vi "Handle UNREGISTERED.vi"(8 "error in (no error)":errorcluster, 9 "WAMP Message":T16 {"Message Codes" items=["HELLO"=1, "WELCOME"=2, "ABORT"=3, "GOODBYE"=6, "ERROR"=8, "PUBLISH"=16, "PUBLISHED"=17, "SUBSCRIBE"=32, "SUBSCRIBED"=33, "UNSUBSCRIBE"=34, "UNSUBSCRIBED"=35, "EVENT"=36, "CALL"=48, "RESULT"=59, "REGISTER"=64, "REGISTERED"=65, "UNREGISTER"=66, "UNREGISTERED"=67, "INVOCATION"=68, "YIELD"=70]}, 10 "Message loop data (in)":T1, 11 "reference":refnum<class "WAMP Client.lvclass">) -> (0 "error out":errorcluster, 2 "Message Loop Data (Out)":T1, 3 "reference out":refnum<class "WAMP Client.lvclass">)   [LabVIEW 2020, in "wamplv.lvlib" / "WAMP Client.lvclass"]
uses:
  <vilib>/samangh/wamplv/WAMP Client/WAMP Client.lvclass
  <vilib>/samangh/wamplv/WAMP Client/TypeDef/WAMP Received Message.ctl
  <vilib>/samangh/wamplv/WAMP Message Codes.ctl
  <vilib>/samangh/wamplv/WAMP Client/TypeDef/Message Loop Shift Reg Data.ctl
  <vilib>/samangh/wamplv/WAMP Client/TypeDef/REGISTER Request Data.ctl
  <vilib>/samangh/wamplv/WAMP Client/TypeDef/Success or error.ctl
  <vilib>/samangh/wamplv/WAMP Client/TypeDef/Combined error.ctl
  <vilib>/samangh/wamplv/WAMP Client/TypeDef/WAMP Error Payload.ctl
  <vilib>/samangh/wamplv/WAMP Client/TypeDef/INVOCATION payload.ctl
  <vilib>/samangh/wamplv/WAMP Client/TypeDef/Publish Requests Map.ctl
  <vilib>/samangh/wamplv/WAMP Client/TypeDef/PUBLISH Request Data.ctl
  <vilib>/samangh/wamplv/WAMP Client/TypeDef/PUBLISH Result.ctl
  <vilib>/samangh/wamplv/WAMP Client/TypeDef/Endpoint Data.ctl
  <vilib>/samangh/wamplv/WAMP Client/TypeDef/CALL Request Map.ctl
  <vilib>/samangh/wamplv/WAMP Client/TypeDef/CALL Request Data.ctl
  <vilib>/samangh/wamplv/WAMP Client/TypeDef/RESULT Payload.ctl
  <vilib>/samangh/wamplv/WAMP Client/TypeDef/SUBSCRIBE Requests Map.ctl
  <vilib>/samangh/wamplv/WAMP Client/TypeDef/SUBSCRIBE Request Data.ctl
  <vilib>/samangh/wamplv/WAMP Client/TypeDef/Subscribe Result.ctl
  <vilib>/samangh/wamplv/WAMP Client/TypeDef/Event Payload.ctl
  <vilib>/samangh/wamplv/WAMP Client/TypeDef/Subscriptions Map.ctl
  <vilib>/samangh/wamplv/WAMP Client/TypeDef/Subscription Details.ctl
  <vilib>/samangh/wamplv/WAMP Client/TypeDef/Unsubscribe Requests Map.ctl
  <vilib>/samangh/wamplv/WAMP Client/TypeDef/UNSUBSCRIBE Request Data.ctl
  <vilib>/samangh/wamplv/WAMP Client/TypeDef/UNSUBSCRIBE Result.ctl
  <vilib>/samangh/wamplv/WAMP Client/TypeDef/Unregister requests map.ctl
  <vilib>/samangh/wamplv/WAMP Client/TypeDef/Unregister request.ctl
  <vilib>/samangh/wamplv/WAMP Client/WAMP Client.lvclass/WAMP Client.ctl
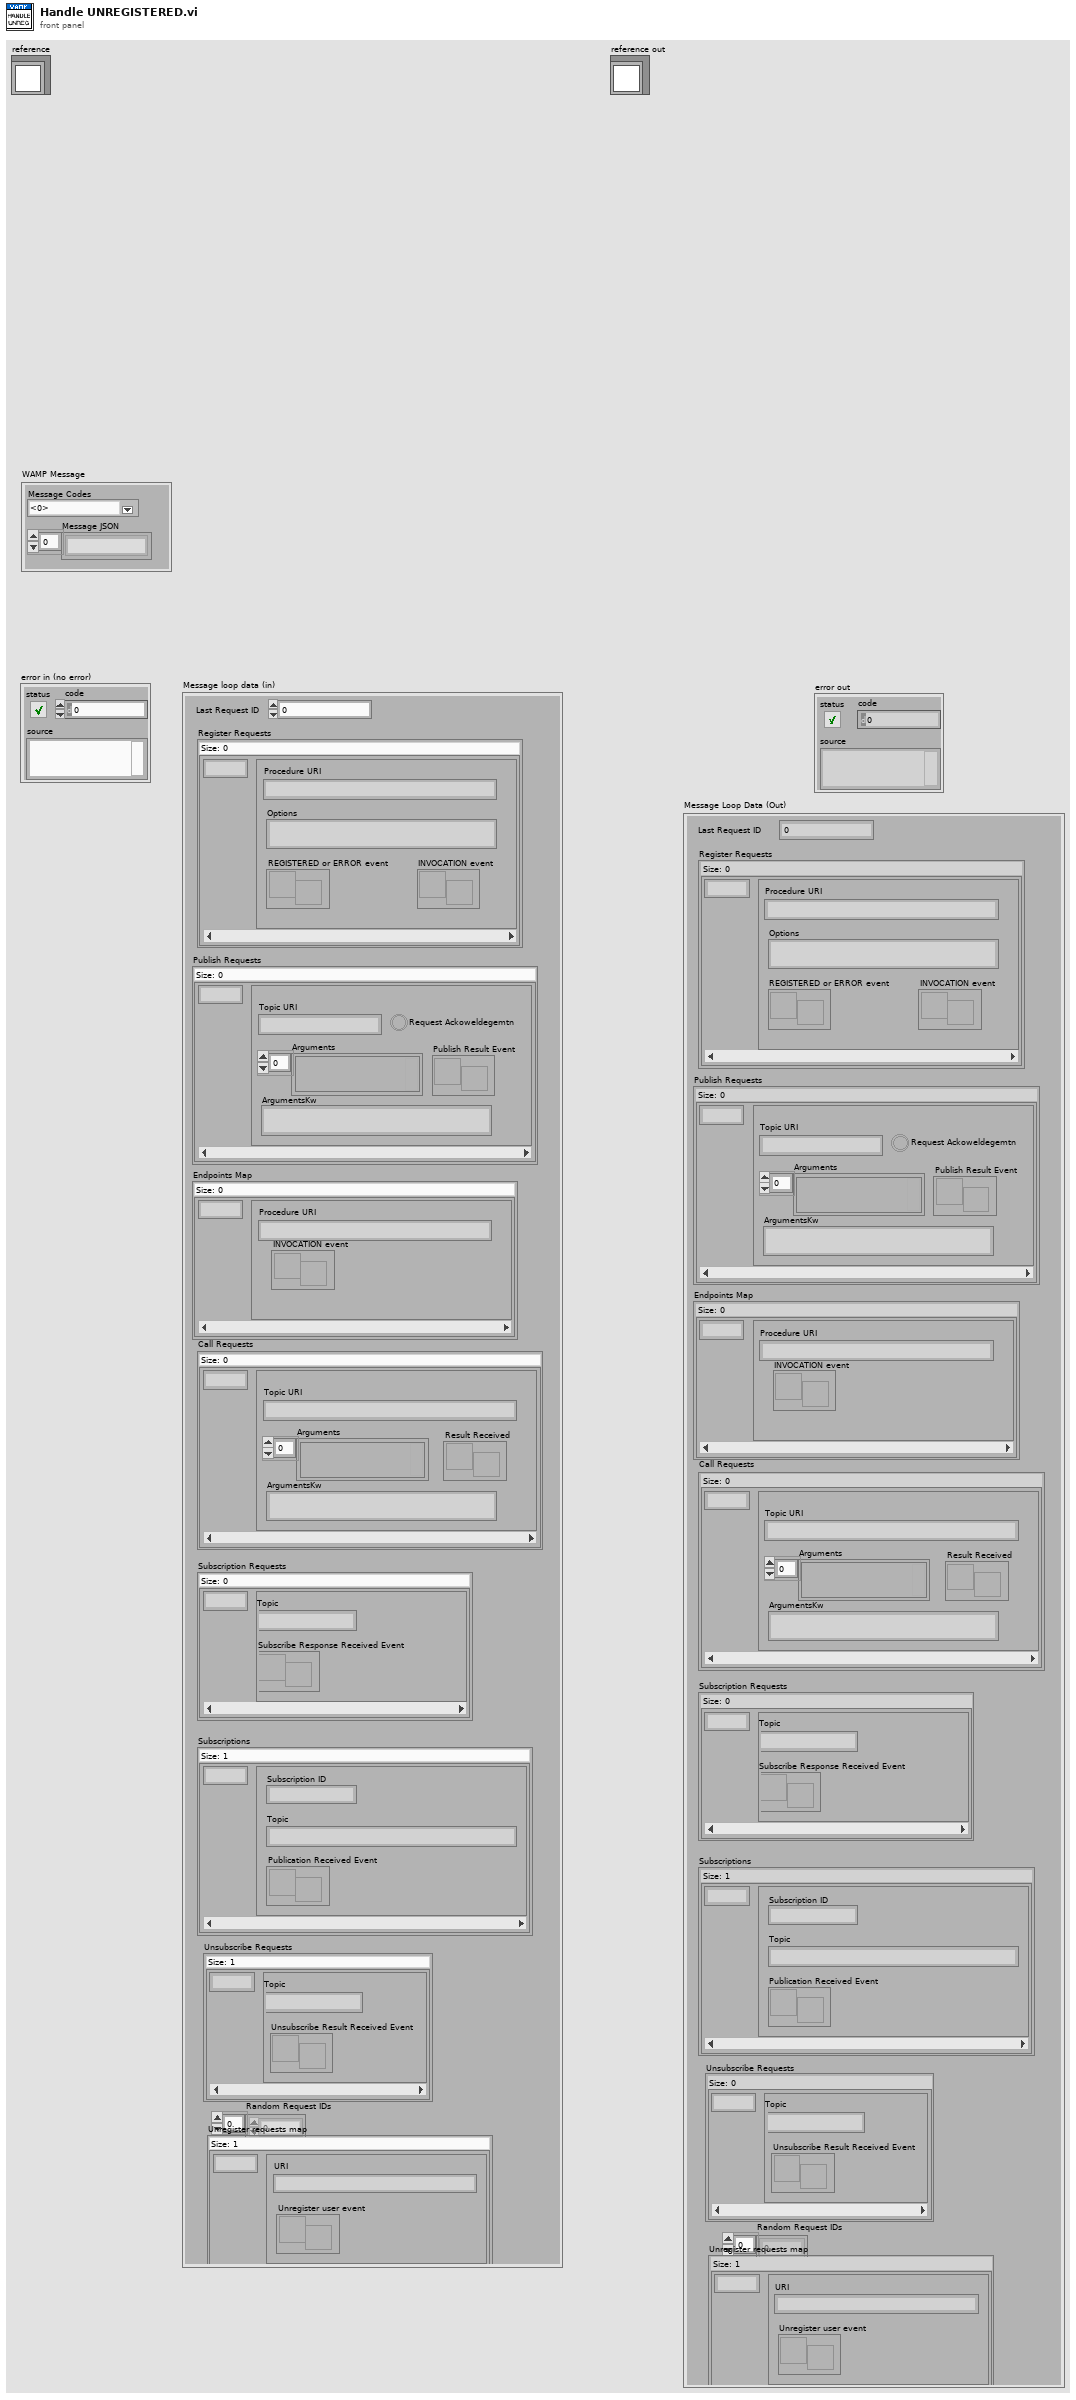
[diagram p1: front panel]
types:
  T1 = typedef "wamplv.lvlib/WAMP Client.lvclass/Message Loop Shift Reg Data.ctl" = cluster{"Last Request ID":u64, "Register Requests":map{u64, T2}, "Publish Requests":T3, "Endpoints Map":map{u64, T5}, "Call Requests":T6, "Subscription Requests":T8, "Subscriptions":T10, "Unsubscribe Requests":T12, "Random Request IDs":u64[], "Unregister requests map":T14}
  T2 = typedef "wamplv.lvlib/WAMP Client.lvclass/REGISTER Request Data.ctl" = cluster{"Procedure URI":string, "Options":string, "REGISTERED or ERROR event":refnum<user-event>, "INVOCATION event":refnum<user-event>}
  T3 = typedef "wamplv.lvlib/WAMP Client.lvclass/Publish Requests Map.ctl" = map{u64, T4}
  T4 = typedef "wamplv.lvlib/WAMP Client.lvclass/PUBLISH Request Data.ctl" = cluster{"Topic URI":string, "Arguments":variant[], "ArgumentsKw":string, "Publish Result Event":refnum<user-event>, "Request Ackoweldegemtn":bool}
  T5 = typedef "wamplv.lvlib/WAMP Client.lvclass/Endpoint Data.ctl" = cluster{"Procedure URI":string, "INVOCATION event":refnum<user-event>}
  T6 = typedef "wamplv.lvlib/WAMP Client.lvclass/CALL Request Map.ctl" = map{u64, T7}
  T7 = typedef "wamplv.lvlib/WAMP Client.lvclass/CALL Request Data.ctl" = cluster{"Topic URI":string, "Arguments":variant[], "ArgumentsKw":string, "Result Received":refnum<user-event>}
  T8 = typedef "wamplv.lvlib/WAMP Client.lvclass/SUBSCRIBE Requests Map.ctl" = map{u64, T9}
  T9 = typedef "wamplv.lvlib/WAMP Client.lvclass/SUBSCRIBE Request Data.ctl" = cluster{"Topic":string, "Subscribe Response Received Event":refnum<user-event>}
  T10 = typedef "wamplv.lvlib/WAMP Client.lvclass/Subscriptions Map.ctl" = map{u64, T11}
  T11 = typedef "wamplv.lvlib/WAMP Client.lvclass/Subscription Details.ctl" = cluster{"Subscription ID":u64, "Topic":string, "Publication Received Event":refnum<user-event>}
  T12 = typedef "wamplv.lvlib/WAMP Client.lvclass/Unsubscribe Requests Map.ctl" = map{u64, T13}
  T13 = typedef "wamplv.lvlib/WAMP Client.lvclass/UNSUBSCRIBE Request Data.ctl" = cluster{"Topic":string, "Unsubscribe Result Received Event":refnum<user-event>}
  T14 = typedef "wamplv.lvlib/WAMP Client.lvclass/Unregister requests map.ctl" = map{u64, T15}
  T15 = typedef "wamplv.lvlib/WAMP Client.lvclass/Unregister request.ctl" = cluster{"URI":string, "Unregister user event":refnum<user-event>}
  T16 = typedef "wamplv.lvlib/WAMP Client.lvclass/WAMP Received Message.ctl" = cluster{"Message JSON":string[], "Message Codes":T17}
  T17 = typedef "wamplv.lvlib/WAMP Client.lvclass/WAMP Message Codes.ctl" = u16
  T18 = typedef "wamplv.lvlib/WAMP Client.lvclass/Success or error.ctl" = cluster{"Success?":bool, "URI":string, "Combined Error":T19}
  T19 = typedef "wamplv.lvlib/WAMP Client.lvclass/Combined error.ctl" = cluster{"Error?":bool, "WAMP Error":T20, "Error":errorcluster}
  T20 = typedef "wamplv.lvlib/WAMP Client.lvclass/WAMP Error Payload.ctl" = cluster{"Details":string, "ArgumentKw Payload":string, "Wamp error?":bool, "Error URI":string, "Arguments Payload":string[]}
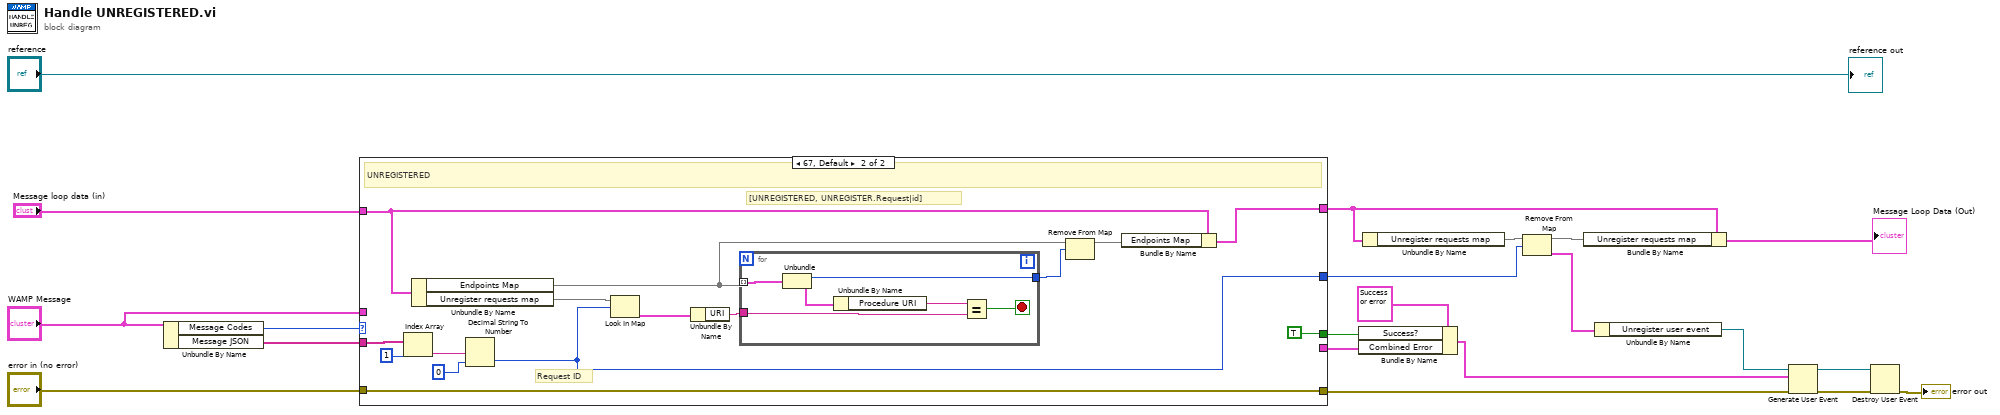
[diagram p0: block diagram]
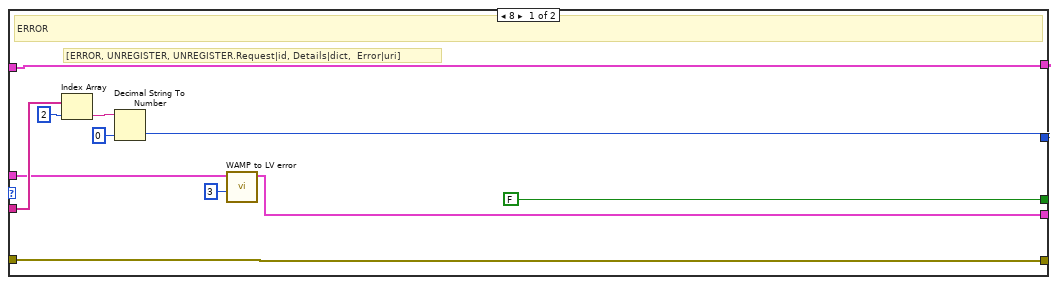
[diagram p2: hidden frame]
diagram:
  n1 = Unbundle By Name("WAMP Message") -> ("Message Codes"=w16:T17, "Message JSON"=w15:string[])
  n2 = case shown="67, Default" w16 {
    tunnel: w15 -> [w30 w46]
    tunnel: [w28 w33] -> w14
    tunnel: "error in (no error)" -> [w29 w45]
    tunnel: [w29 w45] -> w18
    tunnel: [w22 _] -> w20
    tunnel: [FALSE ("Success?") TRUE ("Success?")] -> w19
    tunnel: "Message loop data (in)" -> [w27 w41]
    tunnel: [w27 w40] -> w4
    tunnel: "WAMP Message" -> [w24 _]
    frame 8 {
      # "[ERROR, UNREGISTER, UNREGISTER.Request|id, Details|dict,  Error|uri]"
      # "ERROR"
      n3 = Index Array(array=w30, index=2) -> (element=w31:string)
      n4 = Decimal String To Number(string=w31, default (0L)=u64 0 ("default (0 I32)")) -> (number=w28:u64)  [unwired: 1 in, 1 out]
      n5 = call <vilib>:"WAMP to LV error.vi"("Details Index"=u32 3, "WAMP Message"=w24) -> ("Combined Error"=w22:T19)  [unwired: 7 in, 2 out]
    }
    frame 67, Default {
      # "[UNREGISTERED, UNREGISTER.Request|id]"
      # "Request ID"
      # "UNREGISTERED"
      n6 = Index Array(array=w46, index=1) -> (element=w43:string)
      n7 = Unbundle By Name(w41) -> ("Endpoints Map"=w36:map{u64, T5}, "Unregister requests map"=w37:T14)
      n8 = Decimal String To Number(string=w43, default (0L)=u64 0) -> (number=w33:u64)  [unwired: 1 in, 1 out]
      n9 = Look In Map(map=w37, key=w33) -> (value=w38:T15)  [unwired: 1 in, 1 out]
      n10 = Unbundle By Name(w38) -> ("URI"=w39:string)
      n11 = for {
        tunnel: [w51] -> w34
        tunnel: w36 -> [w49] mode=indexing
        tunnel: w39 -> [w48]
        stop <- w52 stop-if-true
        n12 = Unbundle(w49) -> ("key"=w51:u64, "Endpoint Data"=w53:T5)
        n13 = Unbundle By Name(w53) -> ("Procedure URI"=w50:string)
        n14 = Equal?(x=w50, y=w48) -> (x = y?=w52:bool)
      }
      n15 = Remove From Map(10:w34, 11:w36) -> (3:w35:map{u64, T5})  [unwired: 2 out]
      n16 = Bundle By Name(cluster=w41, "Endpoints Map"=w35) -> (w40:T1)
    }
  }
  n17 = Bundle By Name(cluster=T18 {"Success?"=FALSE, "URI"="", "Combined Error"={"Error?"=FALSE, "WAMP Error"={"Details"="{}", "ArgumentKw Payload"="{}", "Wamp error?"=FALSE, "Error URI"="", "Arguments Payload"=[]}, "Error"={"status"=FALSE, "code"=0, "source"=""}}} ("Sucess or error"), "Success?"=w19, "Combined Error"=w20) -> (w1:T18)
  n18 = Unbundle By Name(w4) -> ("Unregister requests map"=w6:T14)
  n19 = Remove From Map(10:w14, 11:w6) -> (1:w13:T15, 3:w7:T14)  [unwired: 1 out]
  n20 = Bundle By Name(cluster=w4, "Unregister requests map"=w7) -> (→"Message Loop Data (Out)":T1)
  n21 = Unbundle By Name(w13) -> ("Unregister user event"=w9:refnum<user-event>)
  n22 = Generate User Event(user event=w9, event data cluster=w1, error in=w18) -> (user event out=w10:refnum<user-event>, error out=w12:errorcluster)  [unwired: 1 in]
  n23 = Destroy User Event(user event=w10, error in=w12) -> (error out=→"error out":errorcluster)
  "reference out" <- "reference"
